vi "ISX3_Example_ReadDeviceID.vi"() -> ()   [LabVIEW 2012, in "Sciospec ISX3 Impedance Analyzer.lvlib"]
uses:
  Sciospec ISX3 Impedance Analyzer.lvlib
panel:
  out "Number of ISX-3 found":u32
  out "DeviceID of ISX-3":u8[][](array[numeric]) format="%x"
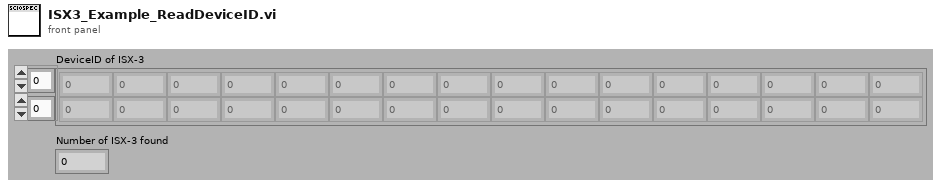
[diagram p1: front panel]
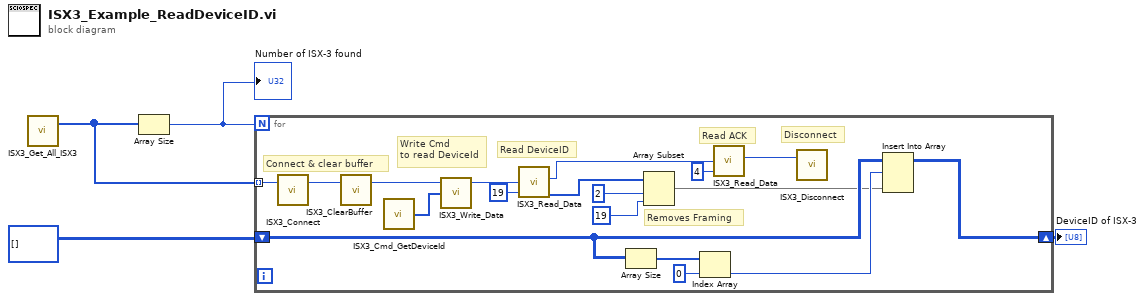
[diagram p0: block diagram]
diagram:
  n1 = call "ISX3_Get_All_ISX3.vi"() -> ("A list of FT_Handel where an ISX-3 is connected to.\nThis handle must be used for further interaction \nwith the USB interface."=w2:u32[])  [unwired: 2 in]
  n2 = Array Size(array=w2) -> (size(s)=w1:i32)
  "Number of ISX-3 found" <- w1
  n3 = for {
    N: w1 -> [_]
    tunnel: w2 -> [w10] mode=indexing
    shift-right: [w15] -> w3
    shift-left: i32[][] [] -> [w18]
    # "Removes Framing"
    # "Connect & clear buffer"
    # "Write Cmd\nto read DeviceId"
    # "Disconnect"
    # "Read ACK"
    # "Read DeviceID"
    n4 = call "ISX3_Connect.vi"("Connect to device with\nFT_Handle"=w10) -> ("Connected to device:"=w5:u32)  [unwired: 2 in]
    n5 = call "ISX3_ClearBuffer.vi"("Handle"=w5) -> ("Handle"=w6:u32)  [unwired: 1 in, 1 out]
    n6 = call "ISX3_Cmd_GetDeviceId.vi"() -> ("DeviceID-Cmd"=w9:u8[])  [unwired: 1 in]
    n7 = call "ISX3_Write_Data.vi"("Data to Write"=w9, "FT_Handle"=w6) -> ("FT_Handle"=w8:u32)  [unwired: 2 in, 1 out]
    n8 = call "ISX3_Read_Data.vi"("FT_Handle"=w8, "Bytes To Read"=u32 19) -> ("Handle"=w11:u32, "Read Data"=w14:u8[])  [unwired: 2 in, 1 out]
    n9 = Array Size(array=w18) -> (size(s)=w17:i32[])
    n10 = Array Subset(array=w14, index=2, length=19) -> (w16:u8[])
    n11 = Index Array(array=w17, index=0) -> (element=w19:i32)
    n12 = call "ISX3_Read_Data.vi"("FT_Handle"=w11, "Bytes To Read"=u32 4) -> ("Handle"=w7:u32)  [unwired: 2 in, 2 out]
    n13 = call "ISX3_Disconnect.vi"("FT_Handle"=w7) -> ()  [unwired: 2 in]
    n14 = Insert Into Array ("In Array einfügen")(array=w18, index (row)=w19, new element=w16) -> (w15:i32[][])  [unwired: 1 in]
  }
  "DeviceID of ISX-3" <- w3
